vi "Get_Named_Serial_Port.vi"(1 "Serial Port Alias":string) -> (0 "Serial Port Name":string)   [LabVIEW 2022 SP3]
uses:
  Anemometry/Anemometry Sub Vis/Globals/Meas_global.vi
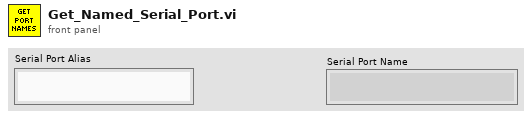
[diagram p1: front panel]
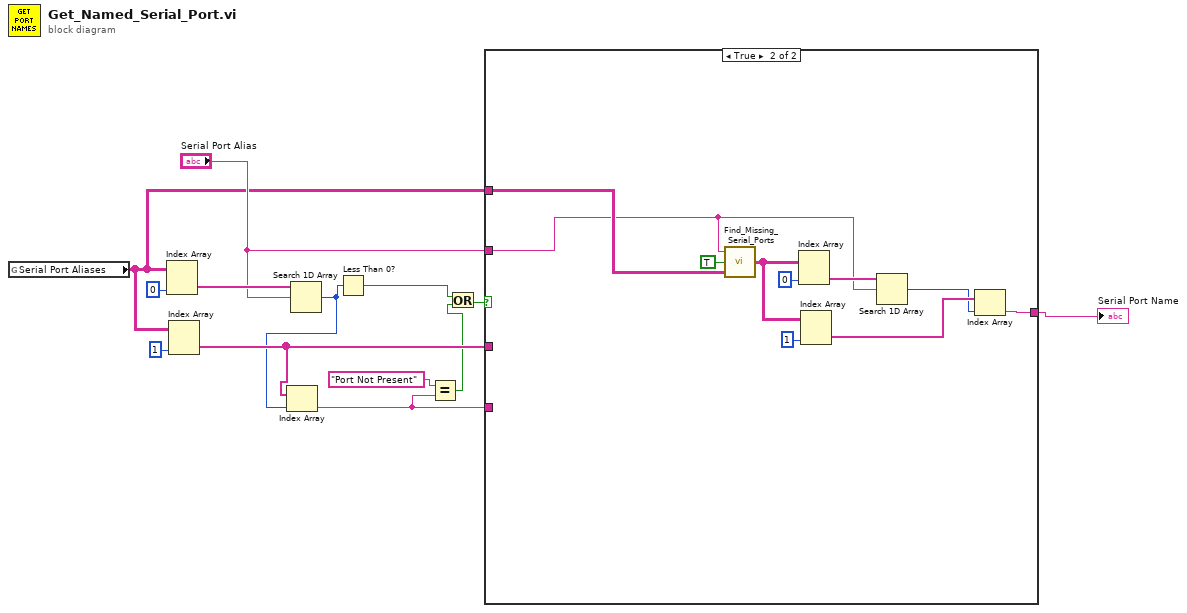
[diagram p0: block diagram]
diagram:
  n1 = global read "Meas_global.vi" "Serial Port Aliases"() -> (w9:string[][])
  n2 = Index Array(array=w9, index (col)=0 ("disabled index (col)")) -> (element=w11:string[])  [unwired: 1 in]
  n3 = Index Array(array=w9, index (col)=1 ("disabled index (col)")) -> (element=w7:string[])  [unwired: 1 in]
  n4 = Search 1D Array(1D array=w11, element="Serial Port Alias") -> (index of element=w6:i32)  [unwired: 1 in]
  n5 = Index Array(array=w7, index=w6) -> (element=w1:string)
  n6 = Less Than 0?(x=w6) -> (x < 0?=w4:bool)
  n7 = Equal?(x="Port Not Present", y=w1) -> (x = y?=w5:bool)
  n8 = Or(x=w4, y=w5) -> (x .or. y?=w3:bool)
  n9 = case shown="True" w3 {
    tunnel: w7 -> [_ _]
    tunnel: "Serial Port Alias" -> [_ w19]
    tunnel: w9 -> [_ w20]
    tunnel: [w14 w16] -> w2
    tunnel: w1 -> [w14 _]
    frame False {
    }
    frame True {
      n10 = call "Find_Missing_Serial_Ports.vi"("Serial Port Aliases"=w20, "Must have Port?"=TRUE, "Aliase to Check"=w19) -> ("Serial Port Aliases Out"=w21:string[][])
      n11 = Index Array(array=w21, index (col)=0 ("disabled index (col)")) -> (element=w22:string[])  [unwired: 1 in]
      n12 = Index Array(array=w21, index (col)=1 ("disabled index (col)")) -> (element=w17:string[])  [unwired: 1 in]
      n13 = Search 1D Array(1D array=w22, element=w19) -> (index of element=w15:i32)  [unwired: 1 in]
      n14 = Index Array(array=w17, index=w15) -> (element=w16:string)
    }
  }
  "Serial Port Name" <- w2
